vi "piezoWriteWriteFuncGen.vi"() -> ()   [LabVIEW 2017]
doc: "Starts the piezo with a triangle or sine wave in continuous mode."
uses:
  <vilib>/DAQmx/write.llb/DAQmx Write (Analog 1D DBL 1Chan NSamp).vi
  globalUtilities.vi
  globalDevices.vi
  <vilib>/DAQmx/miscellaneous.llb/DAQmx Fill In Error Info.vi
panel:
  out "Waveform Graph":dbl[](graph)
  out "used dt":dbl
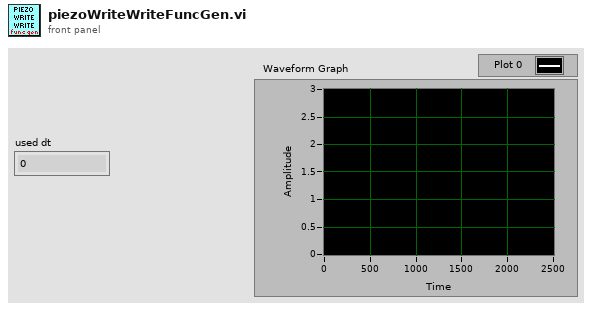
[diagram p1: front panel]
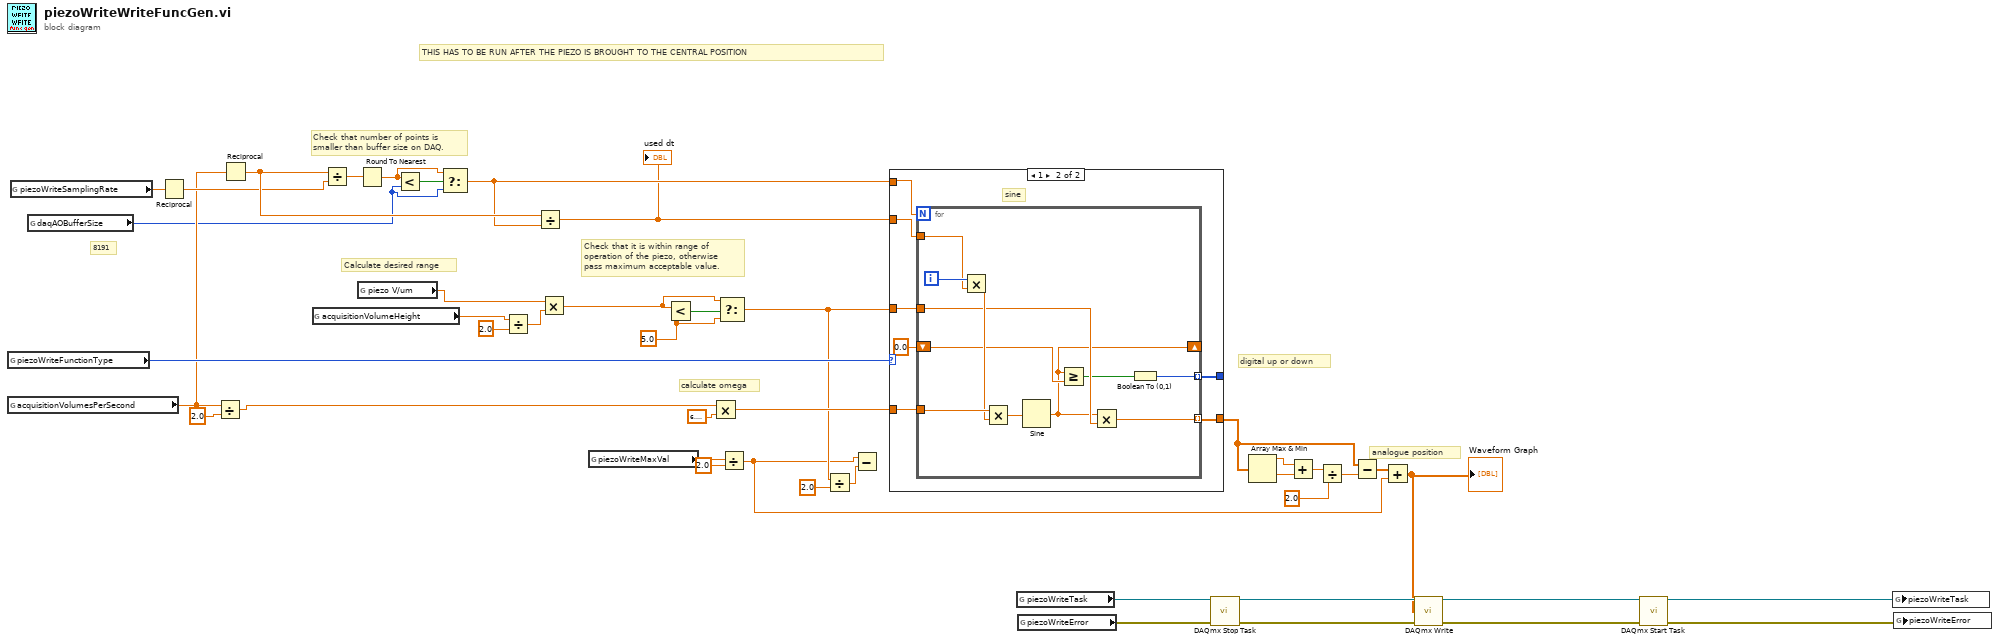
[diagram p0: block diagram]
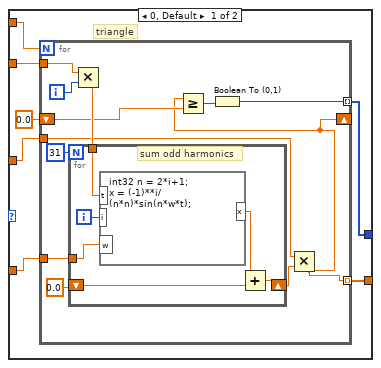
[diagram p2: hidden frame]
diagram:
  w38 = 5.0 ("y")
  # "8191"
  # "analogue position"
  # "digital up or down"
  # "THIS HAS TO BE RUN AFTER THE PIEZO IS BROUGHT TO THE CENTRAL POSITION"
  # "calculate omega"
  # "Check that number of points is\nsmaller than buffer size on DAQ."
  # "Check that it is within range of\noperation of the piezo, otherwise\npass maximum acceptable value."
  # "Calculate desired range"
  n1 = global read "globalDevices.vi" "piezoWriteFunctionType"() -> (w17:u16)
  n2 = global read "globalUtilities.vi" "acquisitionVolumesPerSecond"() -> (w16:dbl)
  n3 = global read "globalDevices.vi" "piezoWriteSamplingRate"() -> (w29:dbl)
  n4 = global read "globalDevices.vi" "daqAOBufferSize"() -> (w13:i32)
  n5 = Reciprocal(x=w29) -> (1/x=w28:dbl)
  n6 = Divide(x=w16, y=2.0) -> (x/y=w14:dbl)
  n7 = Reciprocal(x=w16) -> (1/x=w32:dbl)
  n8 = global read "globalUtilities.vi" "acquisitionVolumeHeight"() -> (w43:dbl)
  n9 = Divide(x=w32, y=w28) -> (x/y=w35:dbl)
  n10 = Round To Nearest(number=w35) -> (nearest integer value=w33:dbl)
  n11 = global read "globalDevices.vi" "piezo V/um"() -> (w44:dbl)
  n12 = Less?(x=w33, y=w13) -> (x < y?=w34:bool)
  n13 = Select(t=w33, s=w34, f=w13) -> (s? t:f=w31:dbl)
  n14 = Divide(x=w43, y=2.0) -> (x/y=w41:dbl)
  n15 = Divide(x=w32, y=w31) -> (x/y=w30:dbl)
  "used dt" <- w30
  n16 = Multiply(x=w44, y=w41) -> (x*y=w39:dbl)
  n17 = global read "globalDevices.vi" "piezoWriteMaxVal"() -> (w27:dbl)
  n18 = Less?(x=w39, y=w38) -> (x < y?=w40:bool)
  n19 = Multiply(x=w14, y=6.283185307179586) -> (x*y=w36:dbl)
  n20 = Select(t=w39, s=w40, f=w38) -> (s? t:f=w11:dbl)
  n21 = Divide(x=w27, y=2.0) -> (x/y=w2:dbl)
  n22 = Divide(x=w11, y=2.0) -> (x/y=w12:dbl)
  n23 = Subtract(x=w2, y=w12) -> ()  [unwired: 1 out]
  n24 = case shown="1" w17 {
    tunnel: w36 -> [w49 w76]
    tunnel: w31 -> [w51 w75]
    tunnel: w30 -> [w50 w74]
    tunnel: w11 -> [w45 w73]
    tunnel: [w48 w72] -> w4
    tunnel: [w46 w70] -> _
    frame 0, Default {
      # "triangle"
      n25 = for {
        N: w51 -> [_]
        tunnel: w50 -> [w63]
        tunnel: w49 -> [w60]
        tunnel: [w52] -> w48 mode=indexing
        shift-right: [w52] -> _
        shift-left: 0.0 -> [w57]
        tunnel: [w55] -> w46 mode=indexing
        tunnel: w45 -> [w54]
        i -> [w62]
        n26 = Multiply(x=w63, y=w62) -> (x*y=w59:dbl)
        n27 = for {
          N: 31 -> [_]
          tunnel: w60 -> [w67]
          tunnel: w59 -> [w69]
          shift-right: [w65] -> w53
          shift-left: 0.0 -> [w64]
          i -> [w68]
          # "sum odd harmonics"
          n28 = formula code="int32 n = 2*i+1;\nx = (-1)**i/(n*n)*sin(n*w*t);"("t"=w69, "i"=w68, "w"=w67) -> ("x"=w66:dbl)
          n29 = Add(x=w66, y=w64) -> (x+y=w65:dbl)
        }
        n30 = Multiply(x=w54, y=w53) -> (x*y=w52:dbl)
        n31 = Greater Or Equal?(x=w52, y=w57) -> (x >= y?=w56:bool)
        n32 = Boolean To (0,1)(Boolean=w56) -> (0, 1=w55:i16)
      }
    }
    frame 1 {
      # "sine"
      n33 = for {
        N: w75 -> [_]
        tunnel: w76 -> [w87]
        tunnel: w74 -> [w85]
        tunnel: w73 -> [w82]
        tunnel: [w77] -> w72 mode=indexing
        shift-right: [w80] -> _
        shift-left: 0.0 -> [w81]
        tunnel: [w78] -> w70 mode=indexing
        i -> [w86]
        n34 = Multiply(x=w86, y=w85) -> (x*y=w84:dbl)
        n35 = Multiply(x=w87, y=w84) -> (x*y=w83:dbl)
        n36 = Sine(x=w83) -> (sin(x)=w80:dbl)
        n37 = Greater Or Equal?(x=w80, y=w81) -> (x >= y?=w79:bool)
        n38 = Multiply(x=w80, y=w82) -> (x*y=w77:dbl)
        n39 = Boolean To (0,1)(Boolean=w79) -> (0, 1=w78:i16)
      }
    }
  }
  n40 = global read "globalDevices.vi" "piezoWriteTask"() -> (w25:refnum<k21>)
  n41 = global read "globalDevices.vi" "piezoWriteError"() -> (w24:errorcluster)
  n42 = call <vilib>:"DAQmx Stop Task.vi"("task/channels in"=w25, "error in"=w24) -> ("task out"=w23:refnum<k21>, "error out"=w22:errorcluster)  [unwired: 12 in]
  n43 = Array Max & Min(array=w4) -> (max value=w9:dbl, min value=w8:dbl)  [unwired: 2 out]
  n44 = Add(x=w9, y=w8) -> (x+y=w7:dbl)
  n45 = Divide(x=w7, y=2.0) -> (x/y=w5:dbl)
  n46 = Subtract(x=w4, y=w5) -> (x-y=w3:dbl[])
  n47 = Add(x=w3, y=w2) -> (x+y=w1:dbl[])
  "Waveform Graph" <- w1
  n48 = call-poly <vilib>:"DAQmx Write.vi"("task/channels in"=w23, "data"=w1, "error in"=w22) -> ("task out"=w19:refnum<k21>, "error out"=w18:errorcluster)  [unwired: 10 in, 1 out]
  n49 = call <vilib>:"DAQmx Start Task.vi"("task/channels in"=w19, "error in"=w18) -> ("task out"=w21:refnum<k21>, "error out"=w20:errorcluster)  [unwired: 12 in]
  n50 = global write "globalDevices.vi" "piezoWriteTask"(w21) -> ()
  n51 = global write "globalDevices.vi" "piezoWriteError"(w20) -> ()
